vi "Teleop.vi"(10 "Match Info":T1={"Autonomous Elapsed Seconds"=0.0, "TeleOp Elapsed Seconds"=0.0, "Disabled Elapsed Seconds"=0.0, "Visited Autonomous"=FALSE, "Visited TeleOp"=FALSE, "Visited Disabled"=FALSE, "Autonomous Settings"={"Autonomous Style"=enum."Independent", "VI Refnum"=refnum}}, 11 "Call Context":T2) -> ()   [LabVIEW 2016]
doc: "This VI is called for each TeleOp packet received from the DS where the robot is not disabled. It is often used to read from the joysticks and update I/O or to update setpoints for timed control loops. It should complete and return within 20 milliseconds or it may miss DS packets."
uses:
  <vilib>/Rock Robotics/WPI/DriverStation/WPI_DriverStationDerivedRobotMode.ctl
  <vilib>/Rock Robotics/WPI/DriverStation/WPI_DriverStationMatch Info.ctl
  <vilib>/Rock Robotics/WPI/Utilities/WPI_GetSetVariantRefNum.vi
  <vilib>/Rock Robotics/Network Tables/NT Write Boolean Array.vi
  <vilib>/Rock Robotics/Network Tables/NT Read Boolean.vi
  <vilib>/Rock Robotics/Network Tables/NT Read Number.vi
  <vilib>/Rock Robotics/Network Tables/NT Write Numeric Array.vi
  <vilib>/Rock Robotics/Network Tables/NT Write Number.vi
panel:
  out "Limited":bool
  in  "Reset Counters":bool
  out "Left + Right OverSpeed":cluster{dbl, dbl}(knob)={10.0, -10.0} scale=-10.0..10.0
  out "Difference":dbl(knob) scale=0.0..50.0
  out "Right Wheel Sensor Count":dbl
  out "Left Wheel Sensor Count":dbl
  out "Sample Slider 0":dbl(slide) scale=0.0..5.0
  out "Sample Boolean 1":bool
  out "Sample Boolean 0":bool
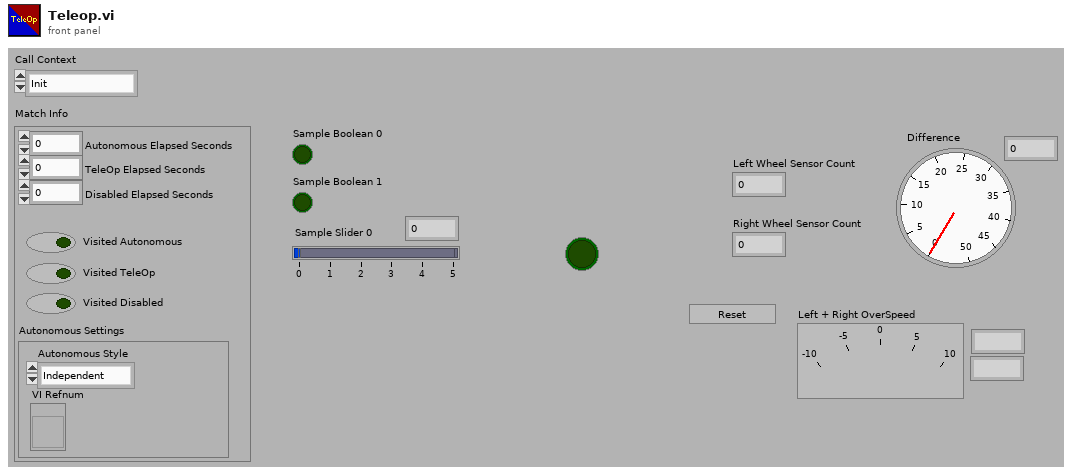
[diagram p1: front panel]
types:
  T1 = typedef "WPI_DriverStationMatch Info.ctl" = cluster{"Autonomous Elapsed Seconds":dbl, "TeleOp Elapsed Seconds":dbl, "Disabled Elapsed Seconds":dbl, "Visited Autonomous":bool, "Visited TeleOp":bool, "Visited Disabled":bool, "Autonomous Settings":cluster{"Autonomous Style":enum16{"Iterative", "Independent"}, "VI Refnum":refnum<vi>}}
  T2 = typedef "WPI_DriverStationDerivedRobotMode.ctl" = enum16{"Init", "Execute", "Stop"}
  T3 = typedef "WPI_JoystickDevRef.ctl" = cluster{"Device":T4}
  T4 = typedef "WPI_JoystickDeviceEnum.ctl" = enum16{"USB 0", "USB 1", "USB 2", "USB 3", "USB 4", "USB 5"}
  T5 = cluster{"Buttons[0]":bool, "Buttons[1]":bool, "Buttons[2]":bool, "Buttons[3]":bool, "Buttons[4]":bool, "Buttons[5]":bool, "Buttons[6]":bool, "Buttons[7]":bool, "Buttons[8]":bool}
  T6 = typedef "WPI_SwitchDevRef.ctl" = cluster{"DevStatus":errorcluster, "DIO Channel":T7, "CntIndex":T8, "Normally Closed":bool}
  T7 = typedef "FPGA_DIOChannel.ctl" = enum8{"DIO 0", "DIO 1", "DIO 2", "DIO 3", "DIO 4", "DIO 5", "DIO 6", "DIO 7", "DIO 8", "DIO 9", "DIO MXP 0", "DIO MXP 1", "DIO MXP 2", "DIO MXP 3", "DIO MXP 4", "DIO MXP 5", "DIO MXP 6", "DIO MXP 7", "DIO MXP 8", "DIO MXP 9", "DIO MXP 10", "DIO MXP 11", "DIO MXP 12", "DIO MXP 13", "DIO MXP 14", "DIO MXP 15", "SPI Port CS1", "SPI Port CS2", "SPI Port CS3", "SPI Port MISO", "SPI Port MOSI", "Invalid"}
  T8 = typedef "FPGA_CounterCtrSystemIndex.ctl" = enum8{"Ctr 0", "Ctr 1", "Ctr 2", "Ctr 3", "Ctr 4", "Ctr 5", "Ctr 6", "Ctr 7", "Invalid"}
  T9 = cluster{"Axes[0]":dbl, "Axes[1]":dbl, "Axes[2]":dbl, "Axes[3]":dbl, "Axes[4]":dbl, "Axes[5]":dbl, "Axes[6]":dbl, "Axes[7]":dbl, "Axes[8]":dbl}
  T10 = typedef "WPI_MotorControlDeviceRef.ctl" = cluster{"DeviceStatus":errorcluster, "Type":T11, "PWM":cluster{"PWM Channel":T12, "DeadBand":T13}, "CAN":cluster{"Device Number":u8, "SetOutput VI Ref":variant, "GetOutput VI Ref":variant, "Enable VI Ref":variant, "Disable VI Ref":variant, "Data":variant}, "Invert":bool}
  T11 = typedef "WPI_MotorControlType.ctl" = enum16{"PWM", "CAN"}
  T12 = typedef "FPGA_DIOPWMChannel.ctl" = enum8{"PWM 0", "PWM 1", "PWM 2", "PWM 3", "PWM 4", "PWM 5", "PWM 6", "PWM 7", "PWM 8", "PWM 9", "PWM MXP 0", "PWM MXP 1", "PWM MXP 2", "PWM MXP 3", "PWM MXP 4", "PWM MXP 5", "PWM MXP 6", "PWM MXP 7", "PWM MXP 8", "PWM MXP 9", "Invalid"}
  T13 = typedef "WPI_PWMDeadband.ctl" = cluster{"Name":string, "maxPositivePwm":i32, "minPositivePwm":i32, "centerPwm":i32, "maxNegativePwm":i32, "minNegativePwm":i32, "angularRange":u16}
  T14 = typedef "WPI_CounterDevRef.ctl" = cluster{"DevStatus":errorcluster, "CntIndex":T8}
  T15 = typedef "WPI_RobotDriveDevRef.ctl" = cluster{"DevStatus":errorcluster, "Motors[]":T10[], "Square Inputs":bool, "Max Output":dbl}
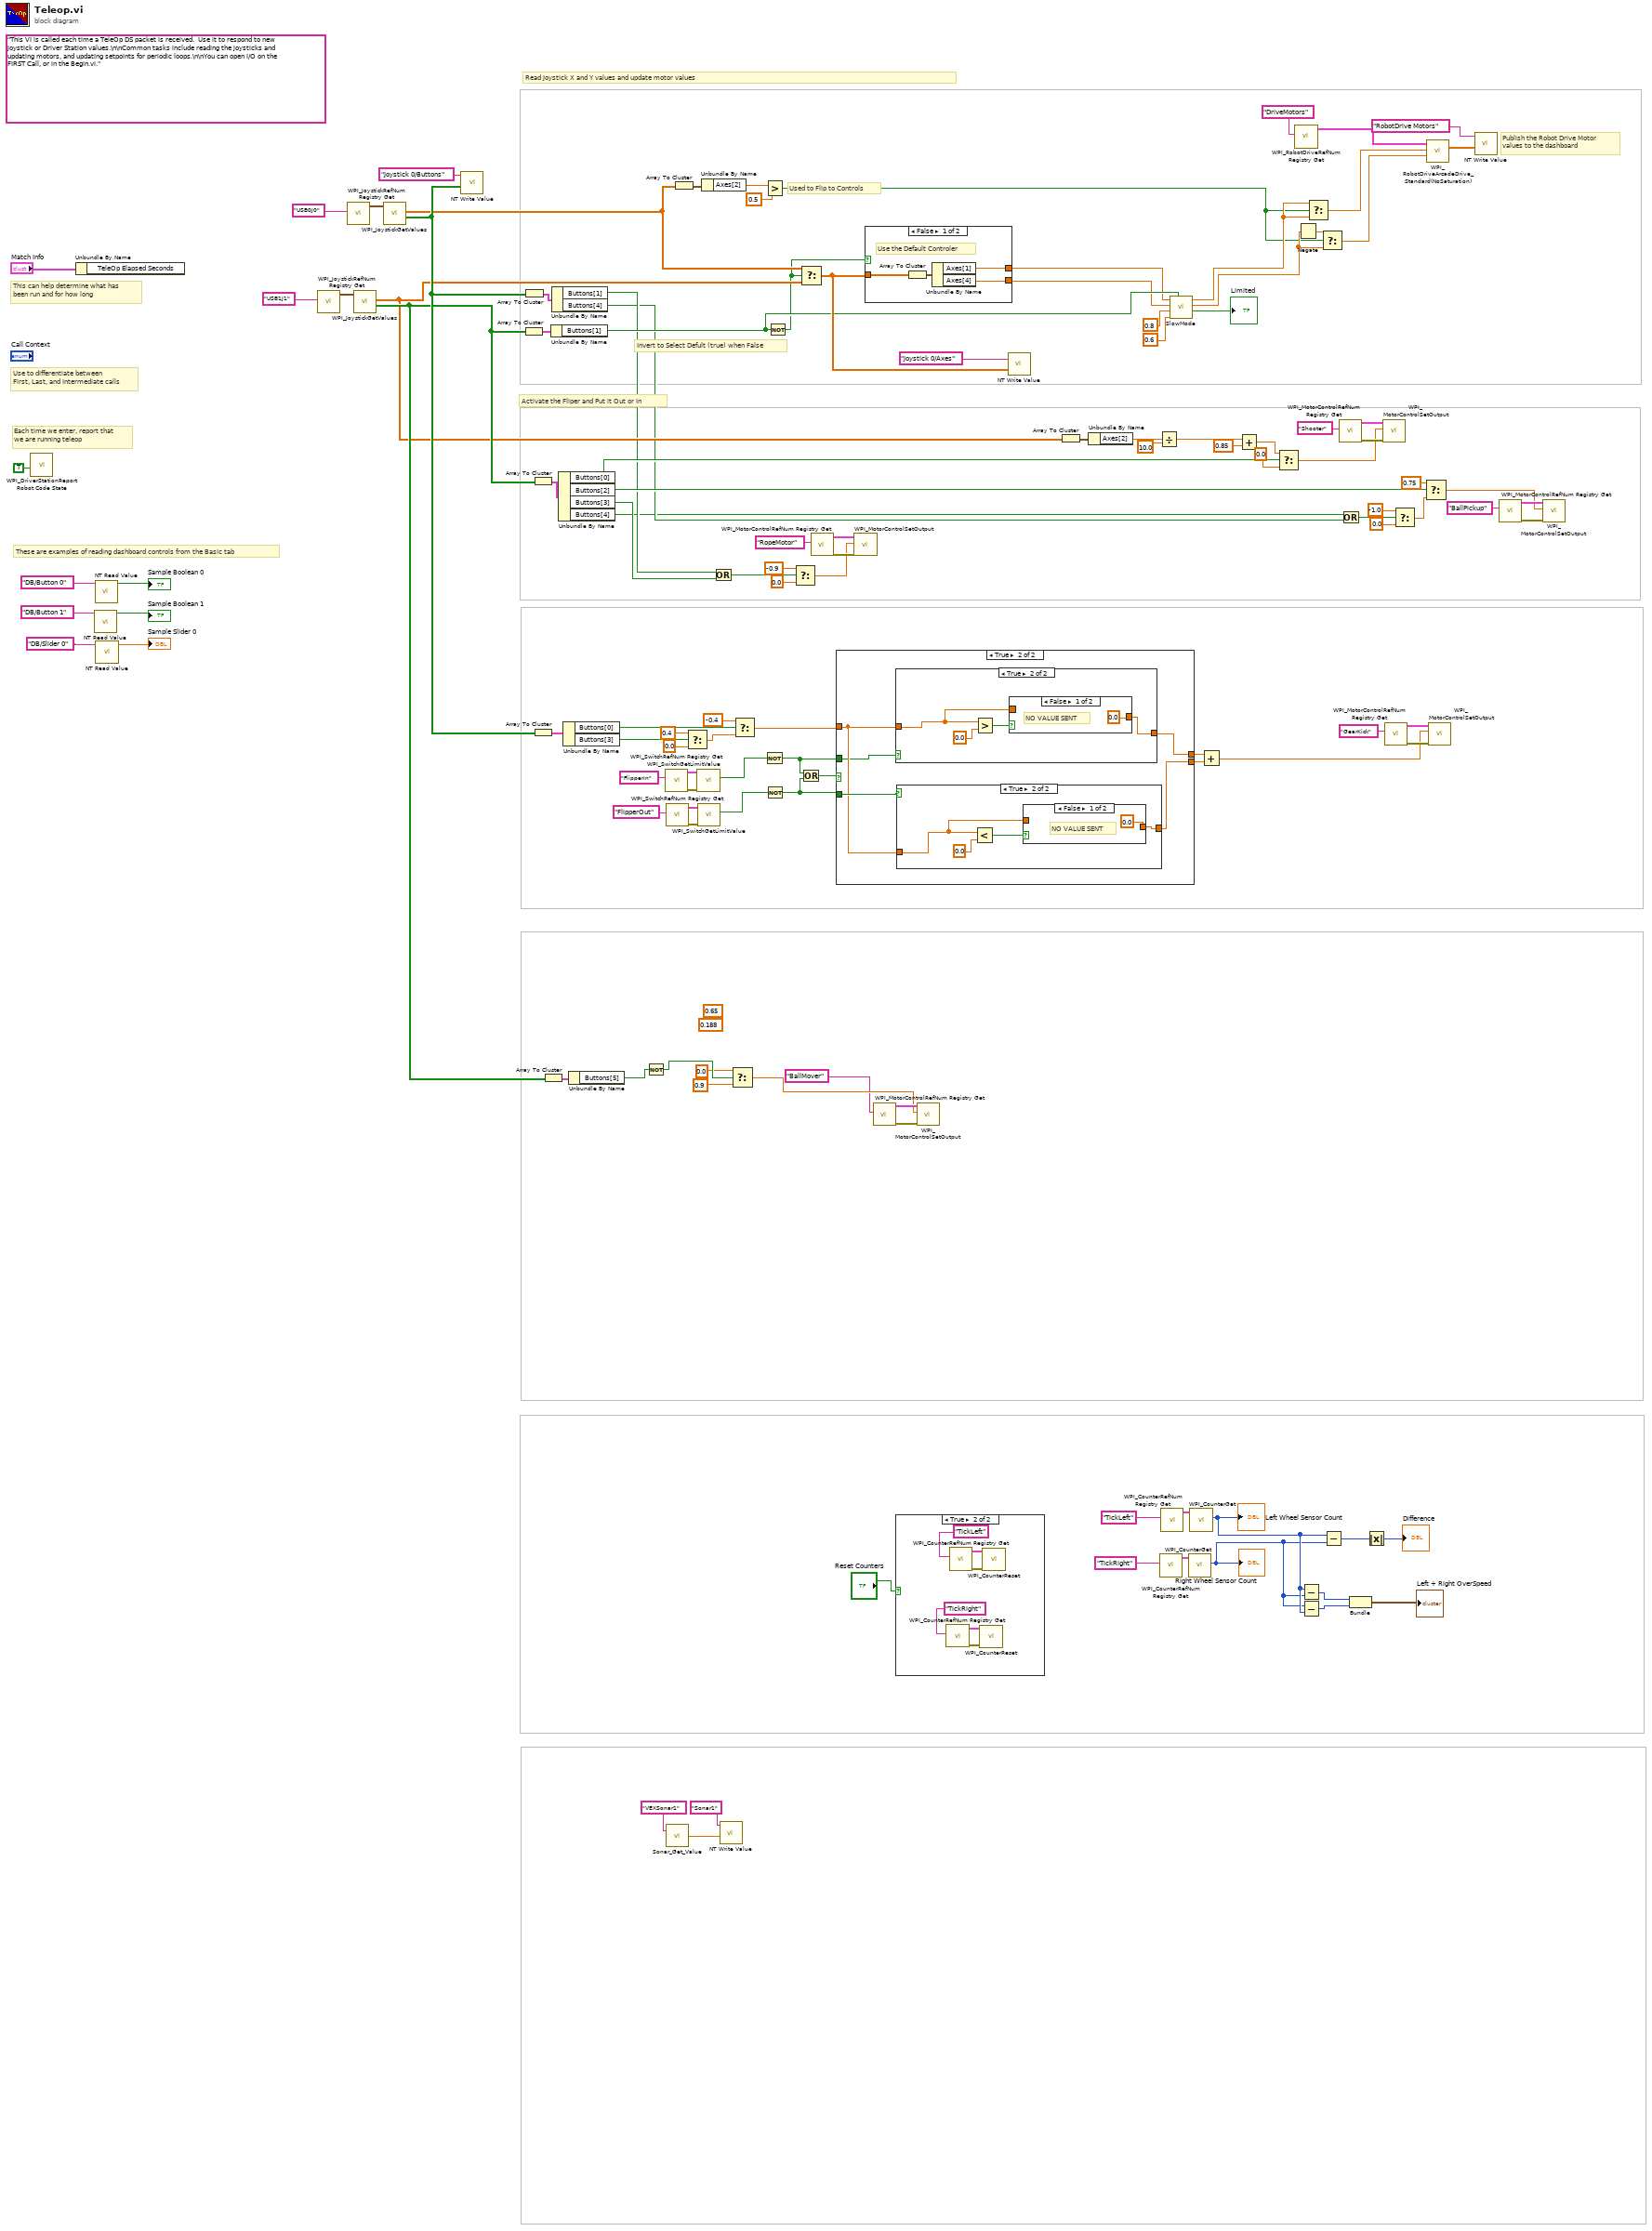
[diagram p0: block diagram]
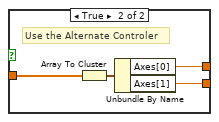
[diagram p2: hidden frame]
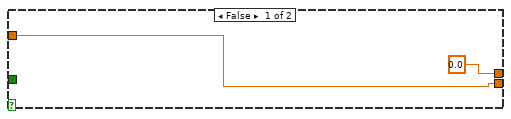
[diagram p4: hidden frame]
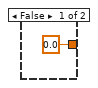
[diagram p5: hidden frame]
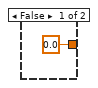
[diagram p7: hidden frame]
diagram:
  (unwired) 0.188 ("f")
  (unwired) 0.65 ("t")
  (unwired) "This VI is called each time a TeleOp DS packet is received.  Use it to respond to new joystick or Driver Station values.\n\nCommon tasks include reading the joysticks and updating motors, and updating setpoints for periodic loops.\n\nYou can open I/O on the FIRST Call, or in the Begin.vi."
  # "Invert to Select Defult (true) when False"
  # "Used to Flip to Controls"
  # "Activate the Fliper and Put it Out or In"
  # "These are examples of reading dashboard controls from the Basic tab"
  # "Publish the Robot Drive Motor\nvalues to the dashboard"
  # "Each time we enter, report that\nwe are running teleop"
  # "Use to differentiate between\nFirst, Last, and Intermediate calls"
  # "This can help determine what has\nbeen run and for how long"
  # "Read Joystick X and Y values and update motor values"
  n1 = call <vilib>:"WPI_DriverStationReport Robot Code State.vi"("TeleOp"=TRUE ("Autonomous")) -> ()  [unwired: 10 in, 1 out]
  n2 = Unbundle By Name("Match Info") -> ()  [unwired: 1 out]
  n3 = call-poly <vilib>:"NT Read Value.vi"("Name"="DB/Button 1" ("refnum name")) -> ("Boolean"=→"Sample Boolean 1":bool)  [unwired: 9 in, 1 out]
  n4 = call-poly <vilib>:"NT Read Value.vi"("Name"="DB/Button 0" ("refnum name")) -> ("Boolean"=→"Sample Boolean 0":bool)  [unwired: 9 in, 1 out]
  n5 = call-poly <vilib>:"NT Read Value.vi"("Name"="DB/Slider 0" ("refnum name")) -> ("Numeric"=→"Sample Slider 0":dbl)  [unwired: 9 in, 1 out]
  n6 = call <vilib>:"WPI_JoystickRefNum Registry Get.vi"("refnum name"="USB1J1") -> ("JoystickDevRef"=w106:T3)  [unwired: 1 in, 9 out]
  n7 = call <vilib>:"WPI_JoystickRefNum Registry Get.vi"("refnum name"="USB0J0") -> ("JoystickDevRef"=w120:T3)  [unwired: 1 in, 9 out]
  n8 = call <vilib>:"WPI_JoystickGetValues.vi"("JoystickDevRef"=w106) -> ("Buttons"=w48:bool[], "Axes"=w22:dbl[])  [unwired: 6 in, 3 out]
  n9 = call <vilib>:"WPI_JoystickGetValues.vi"("JoystickDevRef"=w120) -> ("Buttons"=w57:bool[], "Axes"=w51:dbl[])  [unwired: 6 in, 3 out]
  n10 = call-poly <vilib>:"NT Write Value.vi"("Boolean Array"=w57, "Name"="Joystick 0/Buttons") -> ()  [unwired: 9 in, 1 out]
  n11 = Array To Cluster(array=w48) -> (cluster=w99:T5)
  n12 = Array To Cluster(array=w57) -> (cluster=w58:T5)
  n13 = Array To Cluster(array=w48) -> (cluster=w108:T5)
  n14 = Array To Cluster(array=w57) -> (cluster=w70:T5)
  n15 = Array To Cluster(array=w48) -> (cluster=w49:T5)
  n16 = Unbundle By Name(w99) -> ("Buttons[1]"=w35:bool)
  n17 = Unbundle By Name(w58) -> ("Buttons[1]"=w8:bool, "Buttons[4]"=w6:bool)
  n18 = Unbundle By Name(w108) -> ("Buttons[0]"=w100:bool, "Buttons[2]"=w93:bool, "Buttons[3]"=w7:bool, "Buttons[4]"=w5:bool)
  n19 = Unbundle By Name(w70) -> ("Buttons[0]"=w68:bool, "Buttons[3]"=w69:bool)
  n20 = Unbundle By Name(w49) -> ("Buttons[5]"=w26:bool)
  n21 = Not(x=w26) -> (.not. x?=w17:bool)
  n22 = call <vilib>:"WPI_SwitchRefNum Registry Get.vi"("refnum name"="FlipperIn") -> ("error out"=w78:errorcluster, "SwitchDevRef"=w79:T6)  [unwired: 9 in]
  n23 = call <vilib>:"WPI_SwitchRefNum Registry Get.vi"("refnum name"="FlipperOut") -> ("error out"=w75:errorcluster, "SwitchDevRef"=w76:T6)  [unwired: 9 in]
  n24 = call "Sonar_Get_Value.vi"("RefName"="VEXSonar1") -> ("Inches Out"=w2:dbl)  [unwired: 1 in, 2 out]
  n25 = Array To Cluster(array=w51) -> (cluster=w52:T9)
  n26 = Select(t=0.4, s=w69, f=0.0) -> (s? t:f=w66:dbl)
  n27 = call <vilib>:"WPI_SwitchGetLimitValue.vi"("error in (no error)"=w78, "SwitchDevRef"=w79) -> ("Switch Pressed"=w61:bool)  [unwired: 7 in, 2 out]
  n28 = call <vilib>:"WPI_SwitchGetLimitValue.vi"("error in (no error)"=w75, "SwitchDevRef"=w76) -> ("Switch Pressed"=w62:bool)  [unwired: 7 in, 2 out]
  n29 = Unbundle By Name(w52) -> ("Axes[2]"=w50:dbl)
  n30 = Or(x=w8, y=w7) -> (x .or. y?=w9:bool)
  n31 = call-poly <vilib>:"NT Write Value.vi"("Numeric"=w2, "Name"="Sonar1") -> ()  [unwired: 9 in, 1 out]
  n32 = Select(t=0.0, s=w17, f=0.9) -> (s? t:f=w13:dbl)
  n33 = Select(t=-0.4, s=w68, f=w66) -> (s? t:f=w63:dbl)
  n34 = Not(x=w61) -> (.not. x?=w60:bool)
  n35 = Greater?(x=w50, y=0.5) -> (0:w10:bool)
  n36 = Not(x=w62) -> (.not. x?=w59:bool)
  n37 = Not(x=w35) -> (.not. x?=w4:bool)
  n38 = Select(t=-0.9, s=w9, f=0.0) -> (s? t:f=w89:dbl)
  n39 = Select(t=w51, s=w4, f=w22) -> (s? t:f=w54:dbl[])
  n40 = Or(x=w60, y=w59) -> (x .or. y?=w80:bool)
  n41 = call <vilib>:"WPI_MotorControlRefNum Registry Get.vi"("refnum name"="RopeMotor") -> ("error out"=w92:errorcluster, "MotorControlDevRef"=w91:T10)  [unwired: 9 in]
  n42 = case shown="True" w80 {
    tunnel: w60 -> [_ w129]
    tunnel: w59 -> [_ w131]
    tunnel: w63 -> [w125 w130]
    tunnel: [0.0 ("Axes[1]") w128] -> w73
    tunnel: [w125 w127] -> w72
    frame False {
    }
    frame True {
      n43 = case shown="True" w129 {
        tunnel: w130 -> [_ w141]
        tunnel: [0.0 ("Axes[1]") w140] -> w128
        frame False {
        }
        frame True {
          n44 = Greater?(x=w141, y=0.0) -> (0:w142:bool)
          n45 = case shown="False" w142 {
            tunnel: [0.0 ("Axes[1]") w145] -> w140
            tunnel: w141 -> [_ w145]
            frame False {
              # "NO VALUE SENT"
            }
            frame True {
            }
          }
        }
      }
      n46 = case shown="True" w131 {
        tunnel: w130 -> [_ w133]
        tunnel: [0.0 ("Axes[1]") w134] -> w127
        frame False {
        }
        frame True {
          n47 = Less?(x=w133, y=0.0) -> (x < y?=w135:bool)
          n48 = case shown="False" w135 {
            tunnel: [0.0 ("Axes[1]") w138] -> w134
            tunnel: w133 -> [_ w138]
            frame False {
              # "NO VALUE SENT"
            }
            frame True {
            }
          }
        }
      }
    }
  }
  n49 = call <vilib>:"WPI_MotorControlSetOutput.vi"("error in (no error)"=w92, "Output"=w89, "MotorControlDevRef"=w91) -> ()  [unwired: 6 in, 3 out]
  n50 = case shown="False" w4 {
    tunnel: w54 -> [w148 w152]
    tunnel: [w147 w151] -> w34
    tunnel: [w146 w150] -> w33
    frame False {
      # "Use the Default Controler"
      n51 = Array To Cluster(array=w148) -> (cluster=w149:T9)
      n52 = Unbundle By Name(w149) -> ("Axes[1]"=w147:dbl, "Axes[4]"=w146:dbl)
    }
    frame True {
      # "Use the Alternate Controler"
      n53 = Array To Cluster(array=w152) -> (cluster=w153:T9)
      n54 = Unbundle By Name(w153) -> ("Axes[0]"=w151:dbl, "Axes[1]"=w150:dbl)
    }
  }
  n55 = call <vilib>:"WPI_MotorControlRefNum Registry Get.vi"("refnum name"="BallMover") -> ("error out"=w15:errorcluster, "MotorControlDevRef"=w14:T10)  [unwired: 9 in]
  n56 = case shown="True" "Reset Counters" {
    frame False {
    }
    frame True {
      n57 = call <vilib>:"WPI_CounterRefNum Registry Get.vi"("refnum name"="TickRight") -> ("error out"=w158:errorcluster, "CounterDevRef"=w159:T14)  [unwired: 9 in]
      n58 = call <vilib>:"WPI_CounterRefNum Registry Get.vi"("refnum name"="TickLeft") -> ("error out"=w155:errorcluster, "CounterDevRef"=w156:T14)  [unwired: 9 in]
      n59 = call <vilib>:"WPI_CounterReset.vi"("error in (no error)"=w158, "CounterDevRef in"=w159) -> ()  [unwired: 8 in, 2 out]
      n60 = call <vilib>:"WPI_CounterReset.vi"("error in (no error)"=w155, "CounterDevRef in"=w156) -> ()  [unwired: 8 in, 2 out]
    }
  }
  n61 = call <vilib>:"WPI_MotorControlSetOutput.vi"("error in (no error)"=w15, "Output"=w13, "MotorControlDevRef"=w14) -> ()  [unwired: 6 in, 3 out]
  n62 = call-poly <vilib>:"NT Write Value.vi"("Numeric Array"=w54, "Name"="Joystick 0/Axes") -> ()  [unwired: 9 in, 1 out]
  n63 = Array To Cluster(array=w22) -> (cluster=w25:T9)
  n64 = Unbundle By Name(w25) -> ("Axes[2]"=w21:dbl)
  n65 = Divide(x=w21, y=10.0) -> (x/y=w20:dbl)
  n66 = call <vilib>:"WPI_CounterRefNum Registry Get.vi"("refnum name"="TickRight") -> ("CounterDevRef"=w45:T14)  [unwired: 9 in, 1 out]
  n67 = call <vilib>:"WPI_CounterRefNum Registry Get.vi"("refnum name"="TickLeft") -> ("CounterDevRef"=w46:T14)  [unwired: 9 in, 1 out]
  n68 = call "SlowMode.vi"("Enable"=w35, "Max Speed Y"=0.6 ("Max Speed"), "Max Speed X"=0.8, "Y"=w33, "X"=w34) -> ("UsedLimit/Limited"=→"Limited":bool, "YO"=w29:dbl, "XO"=w27:dbl)  [unwired: 2 in, 2 out]
  n69 = call <vilib>:"WPI_CounterGet.vi"("CounterDevRef in"=w45) -> ("Value"=w38:i32)  [unwired: 5 in, 5 out]
  "Right Wheel Sensor Count" <- w38
  n70 = call <vilib>:"WPI_CounterGet.vi"("CounterDevRef in"=w46) -> ("Value"=w39:i32)  [unwired: 5 in, 5 out]
  "Left Wheel Sensor Count" <- w39
  n71 = Add(x=w73, y=w72) -> (x+y=w71:dbl)
  n72 = Add(x=w20, y=0.85 ("t")) -> (x+y=w24:dbl)
  n73 = Select(t=w24, s=w100, f=0.0) -> (s? t:f=w102:dbl)
  n74 = call <vilib>:"WPI_RobotDriveRefNum Registry Get.vi"("refnum name"="DriveMotors") -> ("RobotDriveDevRef"=w122:T15)  [unwired: 1 in, 9 out]
  n75 = Negate(x=w29) -> (-x=w28:dbl)
  n76 = Subtract(x=w39, y=w38) -> (x-y=w41:i32)
  n77 = Subtract(x=w38, y=w39) -> (x-y=w40:i32)
  n78 = Select(t=w27, s=w10, f=w27) -> (s? t:f=w55:dbl)
  n79 = Select(t=w28, s=w10, f=w29) -> (s? t:f=w56:dbl)
  n80 = Subtract(x=w39, y=w38) -> (x-y=w44:i32)
  n81 = call <vilib>:"WPI_MotorControlRefNum Registry Get.vi"("refnum name"="Shooter") -> ("error out"=w105:errorcluster, "MotorControlDevRef"=w104:T10)  [unwired: 9 in]
  n82 = Or(x=w5, y=w6) -> (x .or. y?=w11:bool)
  n83 = Bundle(w41, w40) -> (→"Left + Right OverSpeed":cluster{i32, i32})  [unwired: 1 in]
  n84 = Absolute Value(x=w44) -> (abs(x)=→"Difference":i32)
  n85 = call <vilib>:"WPI_MotorControlSetOutput.vi"("error in (no error)"=w105, "Output"=w102, "MotorControlDevRef"=w104) -> ()  [unwired: 6 in, 3 out]
  n86 = call <vilib>:"WPI_MotorControlRefNum Registry Get.vi"("refnum name"="GearKick") -> ("error out"=w83:errorcluster, "MotorControlDevRef"=w82:T10)  [unwired: 9 in]
  n87 = Select(t=-1.0, s=w11, f=0.0) -> (s? t:f=w84:dbl)
  n88 = Select(t=0.75, s=w93, f=w84) -> (s? t:f=w95:dbl)
  n89 = call <vilib>:"WPI_RobotDriveArcadeDrive_Standard(NoSaturation).vi"("Y axis value"=w56, "X axis value"=w55, "RobotDriveDevRef"=w122) -> ("Motor Values"=w117:dbl[])  [unwired: 1 in, 7 out]
  n90 = call <vilib>:"WPI_MotorControlSetOutput.vi"("error in (no error)"=w83, "Output"=w71, "MotorControlDevRef"=w82) -> ()  [unwired: 6 in, 3 out]
  n91 = call-poly <vilib>:"NT Write Value.vi"("Numeric Array"=w117, "Name"="RobotDrive Motors") -> ()  [unwired: 9 in, 1 out]
  n92 = call <vilib>:"WPI_MotorControlRefNum Registry Get.vi"("refnum name"="BallPickup") -> ("error out"=w98:errorcluster, "MotorControlDevRef"=w97:T10)  [unwired: 9 in]
  n93 = call <vilib>:"WPI_MotorControlSetOutput.vi"("error in (no error)"=w98, "Output"=w95, "MotorControlDevRef"=w97) -> ()  [unwired: 6 in, 3 out]
